vi "LinearSystemLoop_Elevator_Execute.vi"(5 "ElevatorSim_Model _Params":T2={"DCMOTOR_TYPES"=enum."NEO", "Num Motors"=1, "WinchRadias_Meters"=0.75, "mass_Kg"=26.0, "Gearing"=128.0} {"Gearing" format="%#_13g"; "mass_Kg" format="%#_13g"; "WinchRadias_Meters" format="%#_13g"}, 6 "dT_Seconds":dbl=0.02 format="%#_13g", 7 "LinearSystem_Elevator_Ctrl_Params":T1={"Pos Model Std Dev M"=0.2, "Vel Model Std Dev M/S"=0.8, "Pos Meas Std Dev M"=0.02, "Pos Ctrl Tol M"=0.02, "Vel Ctrl Tol M/S"=0.8, "Max Ctrl Out V"=12.0}, 9 "RawHeight PV":dbl, 10 "Speed SP":dbl, 11 "Height SP":dbl) -> (0 "Error":bool, 2 "Kalman Filtered\nHeight":dbl format="%20.3f", 3 "Motor Dmd (CO)":dbl format="%20.3f", 4 "out Linear System Loop":T4)   [LabVIEW 2019, in "Trajectory_Library.lvlib"]
doc: "Model and control an Elevator system using a Kalman FIlter and LQR controller. This is a single call LabVIEW function.\n\nThe Elevator linear system definition is:\n - States\n - position (meters)\n - velocity (meters/sec)\n - Inputs:\n - motor voltage (volts)\n - Outputs:\n - position (meters)\n\nInputs:\n - LinearSystemId Elevator Model -- cluster -- Packed parameters used to create Elevator linear system.\n - LineaarSystem Elevator Ctrl -- cluster -- Packed parameters used by Kalman Filter and LQR to control the system.\n - Height Setpoint -- double -- Desired height (meters)\n - Speed Setpiont -- double -- Desired speed (meters/sec, Default: 0)\n - Raw Height -- double -- Measured height (meters)\n - dT -- double -- Update time (Seconds, Default: 0.02)\n\nOutputs:\n - Motor Dmd - double -- Motor demand (+/- 1.0)\n - Kalman FIltered Height -- double -- Filtered Height (meters)\n - Error -- boolean -- If TRUE an error occured."
uses:
  Trajectory_Library.lvlib
  <vilib>/Analysis/Matrix/Datatypes/RealMatrix.ctl
  <vilib>/Analysis/Matrix/NI_Matrix.lvlib
  TypeDef/LINEAR_SYSTEM.ctl
  TypeDef/LINEAR_QUADRATIC_REGULATOR.ctl
  TypeDef/LINEAR_PLANT_INV_FF.ctl
  TypeDef/KALMAN_FILTER.ctl
  TypeDef/LINEAR_SYSTEM_LOOP.ctl
  Enum/DCMOTOR_TYPES_ENUM.ctl
  TypeDef/LINEAR_SYSTEM_LOOP_ELEVATOR_CTRL_PARAMS.CTL
  TypeDef/LINEAR_SYSTEM_ID_ELEVATOR_MODEL.CTL
panel:
  # "<States,1>"
  # "<FUTURE --- CLAMP TYPE -- For now\nuse Normalize>"
  # "Steady State Gain  \n<States,Outputs>"
  # "State Estimate <Statess,1>"
  # "<States,States>"
  # "<States,Inputs>"
  # "<Outputs,States>"
  # "<Outputs,Inputs>"
  # "<States,1>"
  # "<Inputs,1>"
  # "<States,Inputs>"
  # "<States,States>"
  # "Ref State <States,1>"
  # "Comp and capped \noutput <Inputs,1>"
  # "Controller gain\n<Inputs,States>"
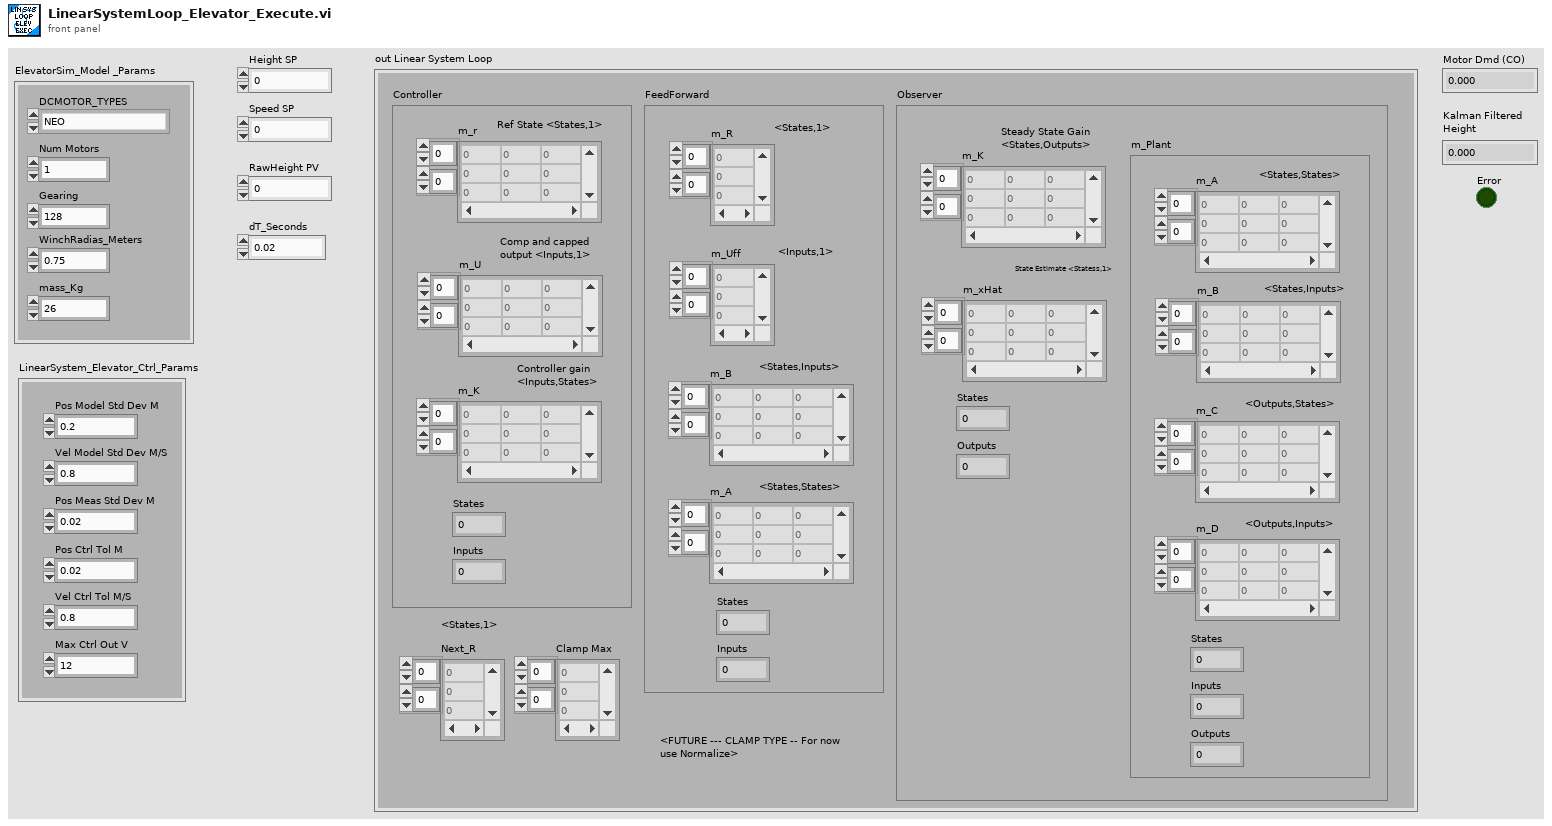
[diagram p1: front panel]
types:
  T1 = typedef "Trajectory_Library.lvlib/LINEAR_SYSTEM_LOOP_ELEVATOR_CTRL_PARAMS.CTL" = cluster{"Pos Model Std Dev M":dbl, "Vel Model Std Dev M/S":dbl, "Pos Meas Std Dev M":dbl, "Pos Ctrl Tol M":dbl, "Vel Ctrl Tol M/S":dbl, "Max Ctrl Out V":dbl}
  T2 = typedef "Trajectory_Library.lvlib/LINEAR_SYSTEM_ID_ELEVATOR_MODEL.CTL" = cluster{"DCMOTOR_TYPES":T3, "Num Motors":i32, "WinchRadias_Meters":dbl, "mass_Kg":dbl, "Gearing":dbl}
  T3 = typedef "Trajectory_Library.lvlib/DCMOTOR_TYPES_ENUM.ctl" = enum16{"CIM", "AndyMark 9015", "Andy Mark RS 775 125", "Bag", "BaneBots RS 550", "BaneBots RS 775", "Falcon 500", "Mini CIM", "NEO", "NEO 550", "Romi BuiltIn", "Vex 775 Pro", "Snow Blower AM 2235A", "Bosch Seat AM 3493", "Falcon 500 FOC", "Kraken X60", "Kraken X60 FOC", "NEO Vortex"}
  T4 = typedef "Trajectory_Library.lvlib/LINEAR_SYSTEM_LOOP.ctl" = cluster{"Controller":T5, "FeedForward":T7, "Observer":T8, "Next_R":T6, "Clamp Max":T6}
  T5 = typedef "Trajectory_Library.lvlib/LINEAR_QUADRATIC_REGULATOR.ctl" = cluster{"m_r":T6, "m_U":T6, "m_K":T6, "States":i32, "Inputs":i32}
  T6 = typedef "NI_Matrix.lvlib/RealMatrix.ctl" = dbl[][]
  T7 = typedef "Trajectory_Library.lvlib/LINEAR_PLANT_INV_FF.ctl" = cluster{"m_R":T6, "m_Uff":T6, "m_B":T6, "m_A":T6, "States":i32, "Inputs":i32}
  T8 = typedef "Trajectory_Library.lvlib/KALMAN_FILTER.ctl" = cluster{"m_K":T6, "m_xHat":T6, "States":i32, "Outputs":i32, "m_Plant":T9}
  T9 = typedef "Trajectory_Library.lvlib/LINEAR_SYSTEM.ctl" = cluster{"m_A":T6, "m_B":T6, "m_C":T6, "m_D":T6, "States":i32, "Inputs":i32, "Outputs":i32}
  T10 = typedef "Trajectory_Library.lvlib/DCMOTOR.CTL" = cluster{"nominalVoltage_Volts":dbl, "StallTorque_NM":dbl, "StallCurrent_Amps":dbl, "FreeCurrent_Amps":dbl, "FreeSpeed_RadPerSec":dbl, "R_Ohms":dbl, "KvINV_RadPerSecPerVolt":dbl, "Kt_NMPerAmp":dbl, "L_H":dbl, "Jr_KgM2":dbl}
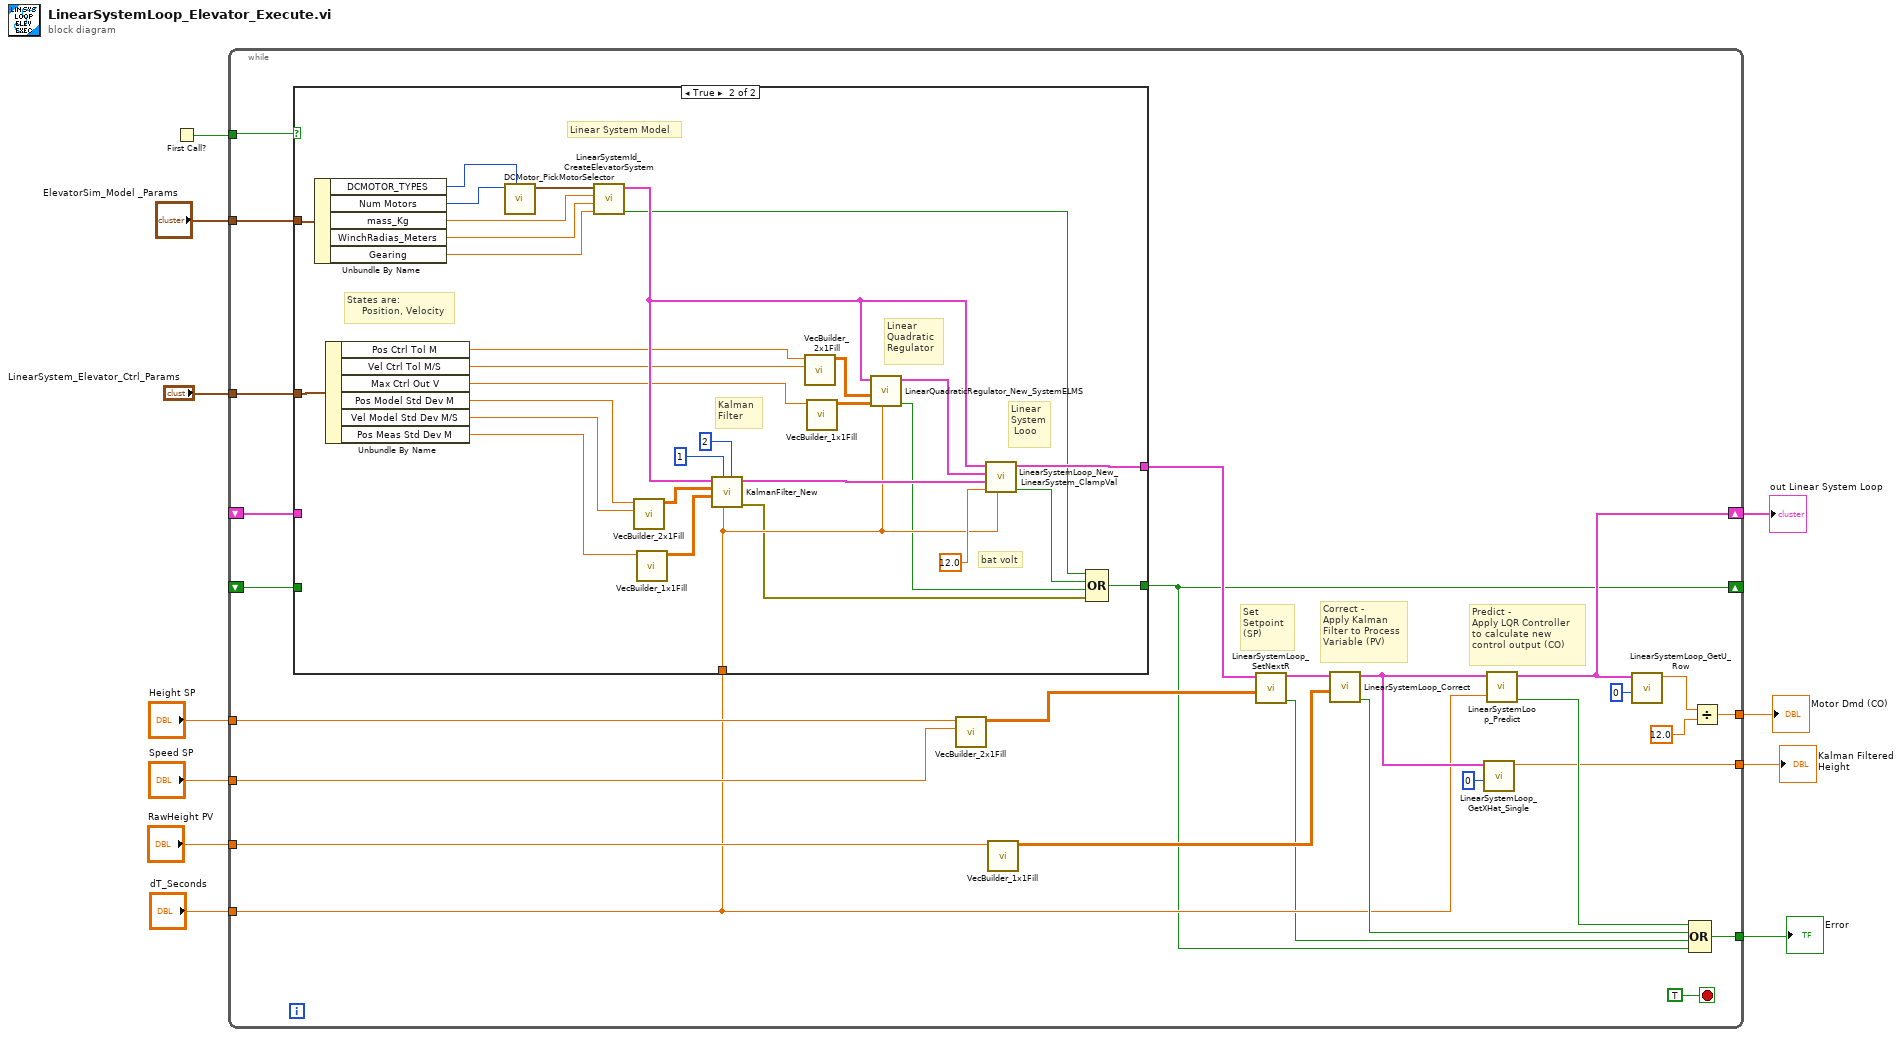
[diagram p0: block diagram]
diagram:
  n1 = First Call?() -> (First Call?: T/F=w3:bool)
  n2 = while {
    tunnel: [w21] -> w11
    tunnel: "dT_Seconds" -> [w18]
    tunnel: [w32] -> w9
    tunnel: "Height SP" -> [w31]
    tunnel: "Speed SP" -> [w30]
    tunnel: "RawHeight PV" -> [w28]
    tunnel: [w24] -> w4
    shift-right: [w27] -> w5
    shift-left: _ -> [w20]
    tunnel: w3 -> [w15]
    tunnel: "ElevatorSim_Model _Params" -> [w17]
    tunnel: "LinearSystem_Elevator_Ctrl_Params" -> [w16]
    shift-right: [w13] -> _
    shift-left: _ -> [w12]
    stop <- TRUE stop-if-true
    # "Predict - \nApply LQR Controller\nto calculate new \ncontrol output (CO)"
    # "Correct - \nApply Kalman\nFilter to Process\nVariable (PV)"
    # "Set\nSetpoint  \n(SP)"
    n3 = case shown="True" w15 {
      tunnel: w20 -> [w40 _]
      tunnel: [w40 w62] -> w19
      tunnel: w18 -> [_ w61]
      tunnel: w17 -> [_ w54]
      tunnel: w16 -> [_ w52]
      tunnel: [w39 w41] -> w13
      tunnel: w12 -> [w39 _]
      frame False {
      }
      frame True {
        # "bat volt"
        # "States are:\n     Position, Velocity"
        # "Linear System Model"
        # "Linear \nSystem\n Looo"
        # "Linear \nQuadratic \nRegulator"
        # "Kalman \nFilter"
        n4 = Unbundle By Name(w54) -> ("DCMOTOR_TYPES"=w59:T3, "Num Motors"=w58:i32, "mass_Kg"=w57:dbl, "WinchRadias_Meters"=w55:dbl, "Gearing"=w56:dbl)
        n5 = Unbundle By Name(w52) -> ("Pos Ctrl Tol M"=w48:dbl, "Vel Ctrl Tol M/S"=w47:dbl, "Max Ctrl Out V"=w46:dbl, "Pos Model Std Dev M"=w51:dbl, "Vel Model Std Dev M/S"=w50:dbl, "Pos Meas Std Dev M"=w49:dbl)
        n6 = call "DCMotor_PickMotorSelector.vi"("DCMOTOR_TYPES"=w59, "Num Motors"=w58) -> ("DCMOTOR"=w60:T10)  [unwired: 9 in]
        n7 = call "LinearSystemId_CreateElevatorSystem.vi"("G"=w56, "radiusMeters"=w55, "massKg"=w57, "DCMOTOR"=w60) -> ("Size Coerced"=w42:bool, "Linearsystem"=w53:T9)  [unwired: 6 in]
        n8 = call "VecBuilder_2x1Fill.vi"("R1"=w50, "R0"=w51) -> ("output matrix"=w67:T6)  [unwired: 9 in]
        n9 = call "VecBuilder_1x1Fill.vi"("R0_C0"=w49) -> ("output matrix"=w68:T6)  [unwired: 10 in]
        n10 = call "KalmanFilter_New.vi"("States"=2, "dt_Seconds"=w61, "Outputs"=1, "MeasurementStdDevs"=w68, "StateStdDevs"=w67, "Plant"=w53) -> ("Error"=w43:errorcluster, "KalmanFilter"=w64:T8)  [unwired: 4 in]
        n11 = call "VecBuilder_2x1Fill.vi"("R1"=w47, "R0"=w48) -> ("output matrix"=w69:T6)  [unwired: 9 in]
        n12 = call "VecBuilder_1x1Fill.vi"("R0_C0"=w46) -> ("output matrix"=w70:T6)  [unwired: 10 in]
        n13 = call "LinearQuadraticRegulator_New_SystemELMS.vi"("dt_Seconds"=w61, "Relms"=w70, "Qelms"=w69, "LINEARSYSTEM"=w53) -> ("Error"=w44:bool, "LinearQuadraticRegulator"=w63:T5)  [unwired: 6 in]
        n14 = call "LinearSystemLoop_New_LinearSystem_ClampVal.vi"("dT_Seconds"=w61, "Max_Voltage"=12.0, "Observer"=w64, "Controller"=w63, "Plant"=w53) -> ("Error"=w45:bool, "Linear System Loop"=w62:T4)  [unwired: 5 in]
        n15 = Compound Arithmetic op=OR(w42, w45, w44, w43) -> (w41:bool)
      }
    }
    n16 = call "VecBuilder_2x1Fill.vi"("R1"=w30, "R0"=w31) -> ("output matrix"=w29:T6)  [unwired: 9 in]
    n17 = call "VecBuilder_1x1Fill.vi"("R0_C0"=w28) -> ("output matrix"=w37:T6)  [unwired: 10 in]
    n18 = call "LinearSystemLoop_SetNextR.vi"("R"=w29, "input inear System Loop"=w19) -> ("Size Coerced"=w14:bool, "out Linear System Loop"=w38:T4)  [unwired: 8 in]
    n19 = call "LinearSystemLoop_Correct.vi"("Y"=w37, "input inear System Loop"=w38) -> ("Error"=w25:bool, "out Linear System Loop"=w36:T4)  [unwired: 8 in]
    n20 = call "LinearSystemLoop_GetXHat_Single.vi"("Row"=0, "input inear System Loop"=w36) -> ("XHat"=w21:dbl)  [unwired: 9 in]
    n21 = call "LinearSystemLoop_Predict.vi"("dT_Seconds"=w18, "input inear System Loop"=w36) -> ("Error"=w26:bool, "out Linear System Loop"=w27:T4)  [unwired: 8 in]
    n22 = call "LinearSystemLoop_GetU_Row.vi"("Row"=0, "input inear System Loop"=w27) -> ("U"=w34:dbl)  [unwired: 9 in]
    n23 = Compound Arithmetic op=OR(w26, w25, w14, w13) -> (w24:bool)
    n24 = Divide(x=w34, y=12.0) -> (x/y=w32:dbl)
  }
  "out Linear System Loop" <- w5
  "Kalman Filtered\nHeight" <- w11
  "Error" <- w4
  "Motor Dmd (CO)" <- w9
